vi "Temperature IR Bricklet Test.vi"() -> ()   [LabVIEW 2011]
uses:
  Classes/Device/Type Definitions/Callback Option.ctl
  Classes/IP Connection/IP Connection.lvclass
  Classes/Device/Device.lvclass
  Classes/Temperature IR Bricklet/Temperature IR Bricklet.lvclass
panel:
  out "appended array":bool[](array[boolean])
  out "x-y":u32
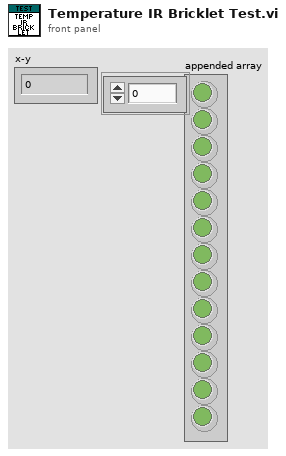
[diagram p1: front panel]
types:
  T1 = typedef "Tinkerforge.lvlib/Device.lvclass/Callback Option.ctl" = enum8{"CB off", "outside range", "inside range", "smaller", "greater"}
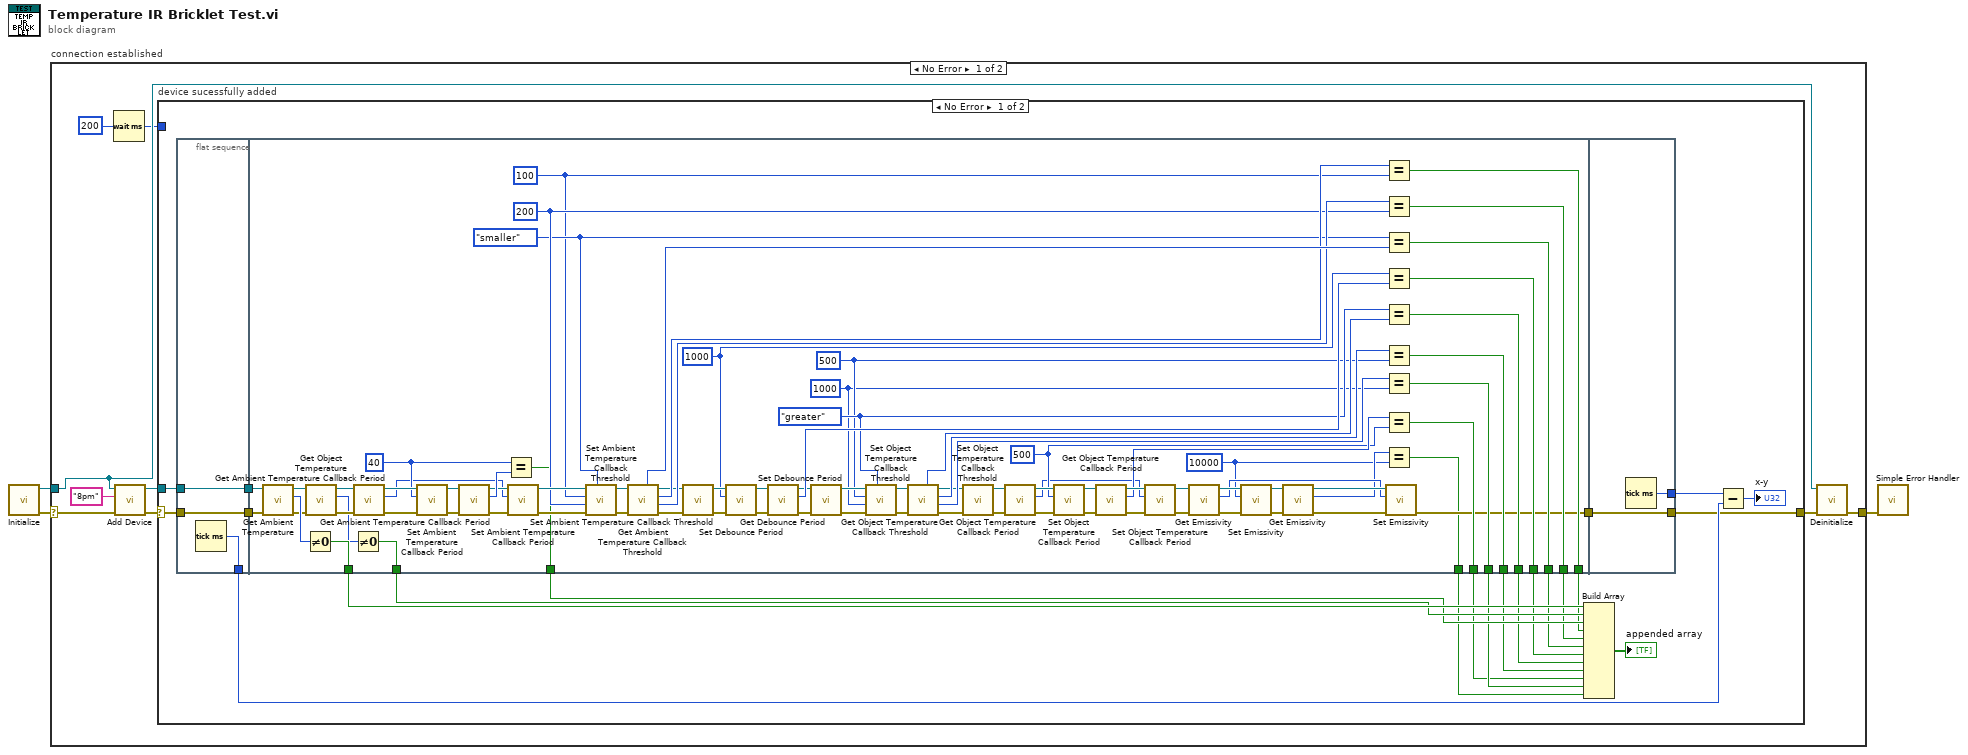
[diagram p0: block diagram]
diagram:
  n1 = call "Initialize.vi"() -> ("error out"=w1:errorcluster, "IP Connection out"=w3:refnum<class "IP Connection.lvclass">)  [unwired: 10 in]
  n2 = case "connection established" shown="No Error" w1 {
    selector: w1 -> [w8 w125]
    tunnel: w3 -> [w12 _]
    tunnel: [w4 w125] -> w2
    frame No Error {
      n3 = Wait (ms)(milliseconds to wait=u32 200) -> (millisecond timer value=w5:u32)
      n4 = call "Add Device.vi"("Error In"=w8, "Device UID"="8pm", "IP Connection"=w12) -> ("Error Out"=w7:errorcluster, "Ambient Light Bricklet"=w9:refnum<class "Temperature IR Bricklet.lvclass">)  [unwired: 7 in]
      n5 = case "device sucessfully added" shown="No Error" w7 {
        selector: w7 -> [w34 w124]
        tunnel: [w14 w124] -> w10
        tunnel: w9 -> [w33 _]
        tunnel: w5 -> [_ _]
        frame No Error {
          n6 = flat-sequence {
            tunnel: w33 -> [w36]
            tunnel: w34 -> [w37]
            tunnel: [w37] -> w31
            tunnel: [w36] -> w30
            tunnel: [w35] -> w28
            tunnel: [w41] -> w32
            tunnel: w31 -> [w121]
            tunnel: w30 -> [w120]
            tunnel: [w66] -> w26
            tunnel: [w65] -> w25
            tunnel: [w64] -> w24
            tunnel: [w63] -> w23
            tunnel: [w62] -> w22
            tunnel: [w61] -> w21
            tunnel: [w60] -> w20
            tunnel: [w59] -> w19
            tunnel: [w58] -> w18
            tunnel: [w57] -> w17
            tunnel: [w56] -> w16
            tunnel: [w38] -> w13
            tunnel: [w123] -> w14
            tunnel: w32 -> [w123]
            tunnel: [w122] -> w29
            frame #0 {
              n7 = Tick Count (ms)() -> (millisecond timer value=w35:u32)
            }
            frame #1 {
              w39 = u16 10000 ("emissivity")
              w68 = u32 500 ("period (0: off)")
              w80 = i16 1000 ("max")
              w82 = i16 500 ("min")
              w85 = Callback_Option."greater" ("Callback Option (off)")
              w95 = u32 1000 ("debounce (100)")
              w103 = i16 200 ("max")
              w88 = i16 100 ("min")
              w89 = Callback_Option."smaller" ("Callback Option (off)")
              w114 = u32 40
              n8 = call "Get Ambient Temperature.vi"("error in (no error)"=w121, "Temperature IR Bricklet in"=w120) -> ("error out"=w55:errorcluster, "Ambient Temperature"=w113:i16, "Temperature IR Bricklet out"=w54:refnum<class "Temperature IR Bricklet.lvclass">)  [unwired: 7 in]
              n9 = Not Equal To 0?(x=w113) -> (x != 0?=w66:bool)
              n10 = call "Get Object Temperature.vi"("error in (no error)"=w55, "Temperature IR Bricklet in"=w54) -> ("error out"=w53:errorcluster, "Object Temperature"=w52:i16, "Temperature IR Bricklet out"=w51:refnum<class "Temperature IR Bricklet.lvclass">)  [unwired: 7 in]
              n11 = Not Equal To 0?(x=w52) -> (x != 0?=w65:bool)
              n12 = call "Get Ambient Temperature Callback Period.vi"("error in (no error)"=w53, "Temperature IR Bricklet in"=w51) -> ("error out"=w119:errorcluster, "period"=w110:u32, "Temperature IR Bricklet out"=w116:refnum<class "Temperature IR Bricklet.lvclass">)  [unwired: 7 in]
              n13 = call "Set Ambient Temperature Callback Period.vi"("error in (no error)"=w119, "period (0: off)"=w114, "Temperature IR Bricklet in"=w116) -> ("error out"=w118:errorcluster, "Temperature IR Bricklet out"=w117:refnum<class "Temperature IR Bricklet.lvclass">)  [unwired: 7 in]
              n14 = call "Get Ambient Temperature Callback Period.vi"("error in (no error)"=w118, "Temperature IR Bricklet in"=w117) -> ("error out"=w112:errorcluster, "period"=w115:u32, "Temperature IR Bricklet out"=w111:refnum<class "Temperature IR Bricklet.lvclass">)  [unwired: 7 in]
              n15 = Equal?(x=w114, y=w115) -> (x = y?=w64:bool)
              n16 = call "Set Ambient Temperature Callback Period.vi"("error in (no error)"=w112, "period (0: off)"=w110, "Temperature IR Bricklet in"=w111) -> ("error out"=w109:errorcluster, "Temperature IR Bricklet out"=w107:refnum<class "Temperature IR Bricklet.lvclass">)  [unwired: 7 in]
              n17 = call "Set Ambient Temperature Callback Threshold.vi"("Callback Option (off)"=w89, "error in (no error)"=w109, "max"=w103, "min"=w88, "Temperature IR Bricklet in"=w107) -> ("error out"=w108:errorcluster, "Temperature IR Bricklet out"=w102:refnum<class "Temperature IR Bricklet.lvclass">)  [unwired: 5 in]
              n18 = call "Get Ambient Temperature Callback Threshold.vi"("error in (no error)"=w108, "Temperature IR Bricklet in"=w102) -> ("error out"=w101:errorcluster, "max"=w104:i16, "min"=w105:i16, "Temperature IR Bricklet out"=w100:refnum<class "Temperature IR Bricklet.lvclass">, "Callback Option"=w106:T1)  [unwired: 5 in]
              n19 = call "Set Ambient Temperature Callback Threshold.vi"("error in (no error)"=w101, "Temperature IR Bricklet in"=w100) -> ("error out"=w99:errorcluster, "Temperature IR Bricklet out"=w98:refnum<class "Temperature IR Bricklet.lvclass">)  [unwired: 8 in]
              n20 = call "Set Debounce Period.vi"("error in (no error)"=w99, "debounce (100)"=w95, "Temperature IR Bricklet in"=w98) -> ("error out"=w96:errorcluster, "Temperature IR Bricklet out"=w97:refnum<class "Temperature IR Bricklet.lvclass">)  [unwired: 7 in]
              n21 = call "Get Debounce Period.vi"("error in (no error)"=w96, "Temperature IR Bricklet in"=w97) -> ("error out"=w93:errorcluster, "debounce"=w94:u32, "Temperature IR Bricklet out"=w92:refnum<class "Temperature IR Bricklet.lvclass">)  [unwired: 7 in]
              n22 = call "Set Debounce Period.vi"("error in (no error)"=w93, "Temperature IR Bricklet in"=w92) -> ("error out"=w91:errorcluster, "Temperature IR Bricklet out"=w90:refnum<class "Temperature IR Bricklet.lvclass">)  [unwired: 8 in]
              n23 = call "Set Object Temperature Callback Threshold.vi"("Callback Option (off)"=w85, "error in (no error)"=w91, "max"=w80, "min"=w82, "Temperature IR Bricklet in"=w90) -> ("error out"=w87:errorcluster, "Temperature IR Bricklet out"=w86:refnum<class "Temperature IR Bricklet.lvclass">)  [unwired: 5 in]
              n24 = call "Get Object Temperature Callback Threshold.vi"("error in (no error)"=w87, "Temperature IR Bricklet in"=w86) -> ("error out"=w79:errorcluster, "max"=w81:i16, "min"=w83:i16, "Temperature IR Bricklet out"=w78:refnum<class "Temperature IR Bricklet.lvclass">, "Callback Option"=w84:T1)  [unwired: 5 in]
              n25 = call "Set Object Temperature Callback Threshold.vi"("error in (no error)"=w79, "Temperature IR Bricklet in"=w78) -> ("error out"=w77:errorcluster, "Temperature IR Bricklet out"=w76:refnum<class "Temperature IR Bricklet.lvclass">)  [unwired: 8 in]
              n26 = call "Get Object Temperature Callback Period.vi"("error in (no error)"=w77, "Temperature IR Bricklet in"=w76) -> ("error out"=w75:errorcluster, "period"=w67:u32, "Temperature IR Bricklet out"=w74:refnum<class "Temperature IR Bricklet.lvclass">)  [unwired: 7 in]
              n27 = call "Set Object Temperature Callback Period.vi"("error in (no error)"=w75, "period (0: off)"=w68, "Temperature IR Bricklet in"=w74) -> ("error out"=w72:errorcluster, "Temperature IR Bricklet out"=w71:refnum<class "Temperature IR Bricklet.lvclass">)  [unwired: 7 in]
              n28 = call "Get Object Temperature Callback Period.vi"("error in (no error)"=w72, "Temperature IR Bricklet in"=w71) -> ("error out"=w70:errorcluster, "period"=w69:u32, "Temperature IR Bricklet out"=w73:refnum<class "Temperature IR Bricklet.lvclass">)  [unwired: 7 in]
              n29 = call "Set Object Temperature Callback Period.vi"("error in (no error)"=w70, "period (0: off)"=w67, "Temperature IR Bricklet in"=w73) -> ("error out"=w50:errorcluster, "Temperature IR Bricklet out"=w49:refnum<class "Temperature IR Bricklet.lvclass">)  [unwired: 7 in]
              n30 = call "Get Emissivity.vi"("error in (no error)"=w50, "Temperature IR Bricklet in"=w49) -> ("error out"=w48:errorcluster, "emissivity"=w42:u16, "Temperature IR Bricklet out"=w47:refnum<class "Temperature IR Bricklet.lvclass">)  [unwired: 7 in]
              n31 = call "Set Emissivity.vi"("error in (no error)"=w48, "emissivity"=w39, "Temperature IR Bricklet in"=w47) -> ("error out"=w45:errorcluster, "Temperature IR Bricklet out"=w44:refnum<class "Temperature IR Bricklet.lvclass">)  [unwired: 7 in]
              n32 = call "Get Emissivity.vi"("error in (no error)"=w45, "Temperature IR Bricklet in"=w44) -> ("error out"=w46:errorcluster, "emissivity"=w40:u16, "Temperature IR Bricklet out"=w43:refnum<class "Temperature IR Bricklet.lvclass">)  [unwired: 7 in]
              n33 = Equal?(x=w105, y=w88) -> (x = y?=w63:bool)
              n34 = Equal?(x=w104, y=w103) -> (x = y?=w62:bool)
              n35 = Equal?(x=w89, y=w106) -> (x = y?=w61:bool)
              n36 = Equal?(x=w95, y=w94) -> (x = y?=w60:bool)
              n37 = Equal?(x=w85, y=w84) -> (x = y?=w59:bool)
              n38 = Equal?(x=w83, y=w82) -> (x = y?=w58:bool)
              n39 = Equal?(x=w81, y=w80) -> (x = y?=w57:bool)
              n40 = Equal?(x=w69, y=w68) -> (x = y?=w56:bool)
              n41 = Equal?(x=w40, y=w39) -> (x = y?=w38:bool)
              n42 = call "Set Emissivity.vi"("error in (no error)"=w46, "emissivity"=w42, "Temperature IR Bricklet in"=w43) -> ("error out"=w41:errorcluster)  [unwired: 7 in, 1 out]
            }
            frame #2 {
              n43 = Tick Count (ms)() -> (millisecond timer value=w122:u32)
            }
          }
          n44 = Build Array(w26, w25, w24, w23, w22, w21, w20, w19, w18, w16, w17, w13) -> (→"appended array":bool[])
          n45 = Subtract(x=w29, y=w28) -> (x-y=→"x-y":u32)
        }
        frame Error {
        }
      }
      n46 = call "Deinitialize.vi"("error in (no error)"=w10, "IP Connection in"=w12) -> ("error out"=w4:errorcluster)  [unwired: 9 in]
    }
    frame Error {
    }
  }
  n47 = call <vilib>:"Simple Error Handler.vi"("error in (no error)"=w2) -> ()  [unwired: 4 in, 5 out]
